vi "ComputeWfmScalar.vi"(6 "GrpCfg":T1, 7 "Speed":T2, 8 "error in (no error)":errorcluster, 10 "Y Array":sgl[](array[numeric]), 11 "Channel in":refnum<class "Channel.lvclass">) -> (0 "error out":errorcluster, 2 "Metric":dbl, 3 "Channel Out":refnum<class "Channel.lvclass">)   [LabVIEW 2018, in "Measurement Channels.lvlib" / "Channel.lvclass"]
uses:
  Channel.lvclass
  Common/Controls/TE_Designator.ctl
  Common/Controls/Group Timing Info.ctl
  <vilib>/Analysis/baseanly.llb/Mean (DBL).vi
  <vilib>/Analysis/NI_AALBase.lvlib
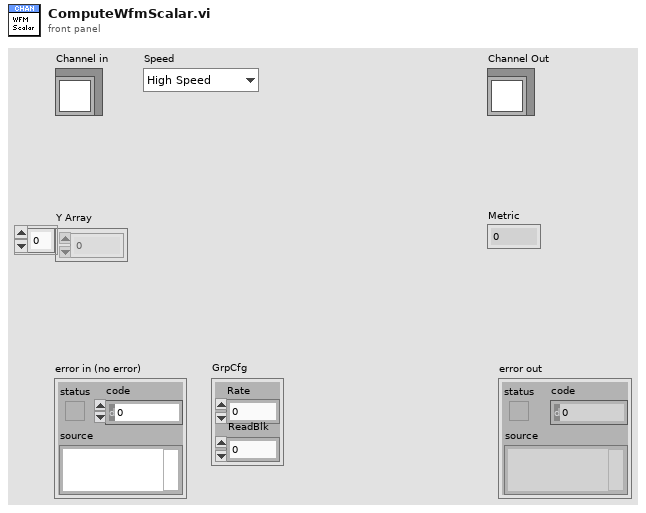
[diagram p1: front panel]
types:
  T1 = typedef "Group Timing Info.ctl" = cluster{"Rate":dbl, "ReadBlk":i32}
  T2 = typedef "TE_Designator.ctl" = enum16{"High Speed", "Low Speed"}
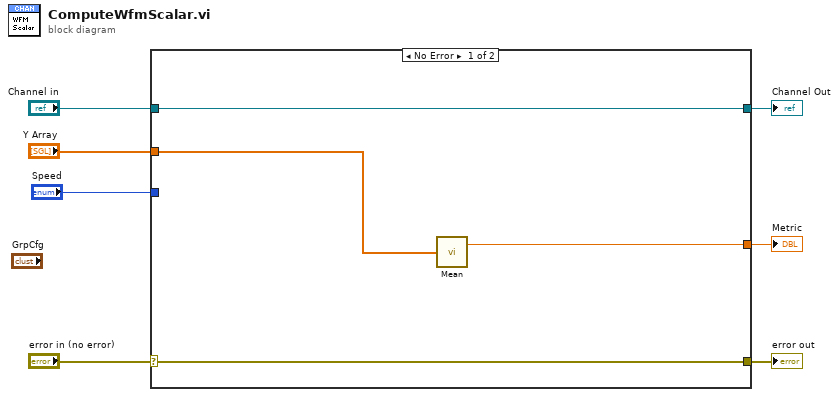
[diagram p0: block diagram]
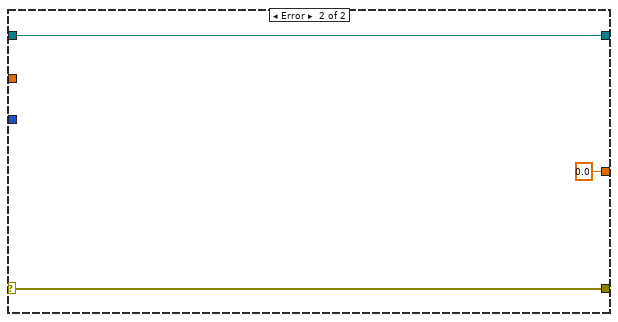
[diagram p2: hidden frame]
diagram:
  n1 = case shown="No Error" "error in (no error)" {
    selector: "error in (no error)" -> [w11 w14]
    tunnel: [w11 w14] -> w6
    tunnel: "Channel in" -> [w10 w12]
    tunnel: "Y Array" -> [w8 _]
    tunnel: "Speed" -> [_ _]
    tunnel: [w9 0.0 ("mean")] -> w2
    tunnel: [w10 w12] -> w1
    frame No Error {
      n2 = call-poly <vilib>:"Mean.vi"("X"=w8) -> ("mean"=w9:dbl)  [unwired: 1 out]
    }
    frame Error {
    }
  }
  "error out" <- w6
  "Metric" <- w2
  "Channel Out" <- w1
